vi "Pop-up wait with progress bar.vi"(8 "error in (no error)":errorcluster, 9 "Prompt Text":string, 10 "Progress (0.0-1.0) in":dbl(slide) scale=0.0..1.0 scale format="%_3f", 11 "Control":enum16{"Open", "Close", "Status", "No Change"}(ring)) -> (0 "error out":errorcluster)   [LabVIEW 2009, in "GUI.lvlib"]
doc: "If there is no error in, this vi will either open or close the calling panel which displays a prompt to wait. The input control determines whether the panel is opened or closed. Typically called before intensive processing with control=open and after with control = close.\n\nClose action ignores error in."
uses:
  GUI.lvlib
  Timing/Timing Lib.lvlib
panel:
  out "Progress (0.0-1.0)":dbl(slide) scale=0.0..1.0 scale format="%_3f"
  out "Prompt":string
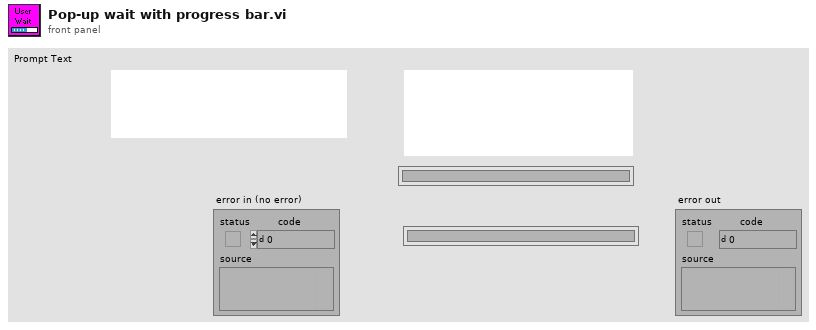
[diagram p1: front panel]
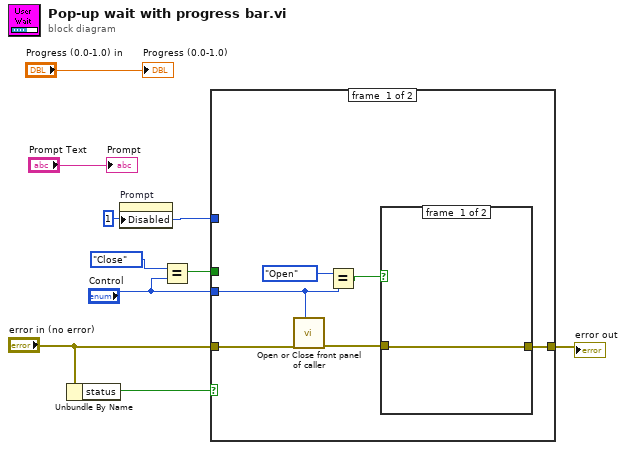
[diagram p0: block diagram]
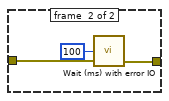
[diagram p2: hidden frame]
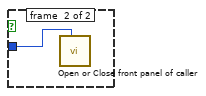
[diagram p4: hidden frame]
diagram:
  w3 = u8 1 ("Write Attribute")
  n1 = Unbundle By Name("error in (no error)") -> ("status"=w7:bool)
  n2 = property on="Prompt" class="Str"("Disabled"=w3) -> ()  [unwired: 2 in, 2 out]
  n3 = Equal?(x=enum16{"Open", "Close", "Status", "No Change"}."Close", y="Control") -> (x = y?=w5:bool)
  n4 = case shown="False" w7 {
    tunnel: [w10 w22] -> w9
    tunnel: "error in (no error)" -> [w15 w22]
    tunnel: w5 -> [_ w21]
    tunnel: "Control" -> [w14 w20]
    tunnel: w3 -> [_ _]
    frame #0 {
      n5 = call "Open or Close front panel of caller.vi"("Control"=w14, "error in (no error)"=w15) -> ("error out"=w11:errorcluster)  [unwired: 4 in, 3 out]
      n6 = Equal?(x=enum16{"Open", "Close", "Status", "No Change"}."Open", y=w14) -> (x = y?=w12:bool)
      n7 = case shown="True" w12 {
        tunnel: w11 -> [w16 w19]
        tunnel: [w16 w18] -> w10
        frame #0 {
        }
        frame #1 {
          n8 = call "Wait (ms) with error IO.vi"("error in (no error)"=w19, "milliseconds to wait"=u32 100) -> ("error out"=w18:errorcluster)  [unwired: 3 in]
        }
      }
    }
    frame #1 {
      n9 = case shown="True" w21 {
        tunnel: w20 -> [_ w23]
        frame #0 {
        }
        frame #1 {
          n10 = call "Open or Close front panel of caller.vi"("Control"=w23) -> ()  [unwired: 5 in, 4 out]
        }
      }
    }
  }
  "error out" <- w9
  "Prompt" <- "Prompt Text"
  "Progress (0.0-1.0)" <- "Progress (0.0-1.0) in"
